vi "nodlltests.vi"() -> ()   [LabVIEW 2017]
panel:
  out "Boolean":bool=TRUE
  out "Meter":dbl(knob) scale=-3.0..3.0
  out "Boolean 3":bool
  out "Boolean 2":bool
  in  "stop":bool
  in  "?":bool
  in  "CW":bool
  in  "Speed":dbl(knob) scale=0.0..3.0
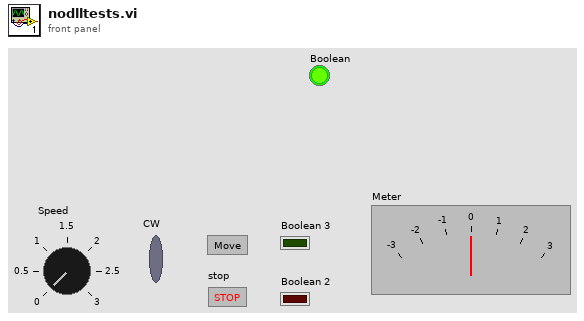
[diagram p1: front panel]
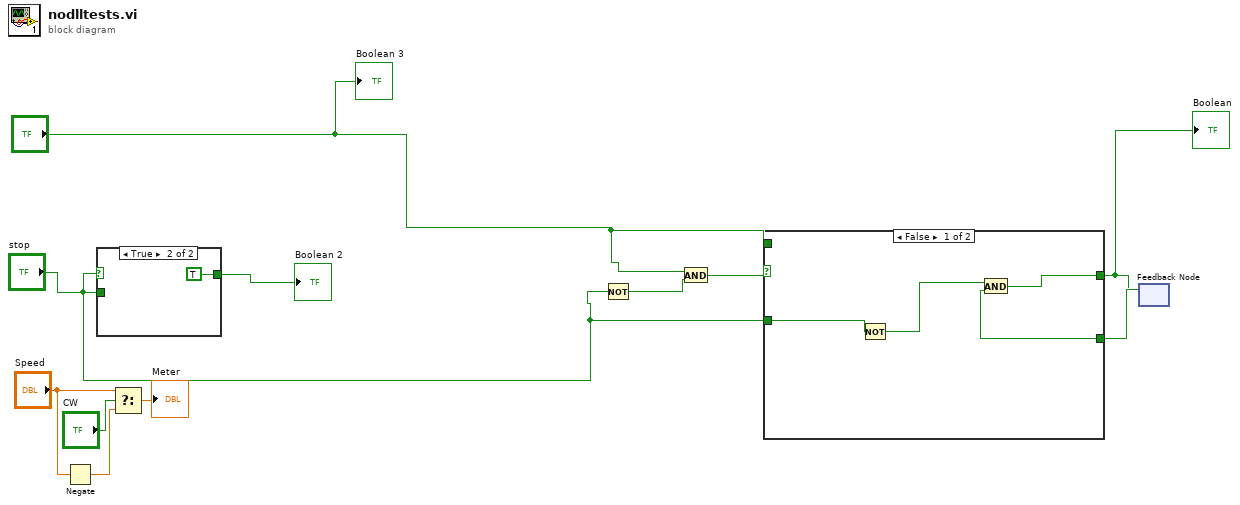
[diagram p0: block diagram]
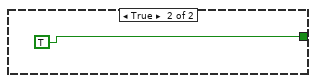
[diagram p2: hidden frame]
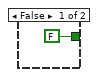
[diagram p3: hidden frame]
diagram:
  n1 = Negate(x="Speed") -> (-x=w11:dbl)
  n2 = case shown="True" "stop" {
    tunnel: "stop" -> [_ _]
    tunnel: [FALSE TRUE] -> w8
    frame False {
    }
    frame True {
    }
  }
  "Boolean 2" <- w8
  n3 = Select(t="Speed", s="CW", f=w11) -> (s? t:f=→"Meter":dbl)
  n4 = Not(x="stop") -> (.not. x?=w6:bool)
  n5 = And(x="?", y=w6) -> (x .and. y?=w5:bool)
  n6 = feedback #1() -> (w2:bool)  [unwired: 1 in]
  n7 = case shown="False" w5 {
    tunnel: [w15 TRUE] -> w1
    tunnel: "?" -> [_ _]
    tunnel: "stop" -> [w17 _]
    tunnel: w2 -> [w14 _]
    frame False {
      n8 = Not(x=w17) -> (.not. x?=w16:bool)
      n9 = And(x=w16, y=w14) -> (x .and. y?=w15:bool)
    }
    frame True {
    }
  }
  "Boolean" <- w1
  n10 = feedback-in #1(w1) -> ()
  "Boolean 3" <- "?"
